vi "Write Evaluations to Limit File.vi"(8 "error in (no error)":errorcluster, 9 "Test Modes":string[](array[string]), 10 "Evaluations In":T1[](array[typedef]) {"Low Limit" format="%#_13g"; "SI Scaling" items=["femto"=-15, "pico"=-12, "nano"=-9, "micro"=-6, "milli"=-3, "percent"=-2, ""=0, "kilo"=3, "mega"=6, "giga"=9, "tera"=12]}, 11 "Limits File Path":path) -> (0 "error out":errorcluster)   [LabVIEW 2018, in "Test Number and Bin Generator.lvlib" / "Test Number and Bin Generator.lvclass"]
uses:
  Test Number and Bin Generator.lvclass
  Plugins/TestStand API Tools (TSAT).lvlibp/Evaluation Actions/Includes/Controls/TSAT Evaluation.ctl
  Plugins/TestStand API Tools (TSAT).lvlibp/Evaluation Actions/Includes/Controls/TSAT Eval SI Unit Scaling.ctl
  Plugins/TestStand API Tools (TSAT).lvlibp/Evaluation Actions/Includes/Controls/TSAT Evaluation Type.ctl
  Plugins/TestStand API Tools (TSAT).lvlibp/Evaluation Actions/TSAT Evaluation Actions.lvlib
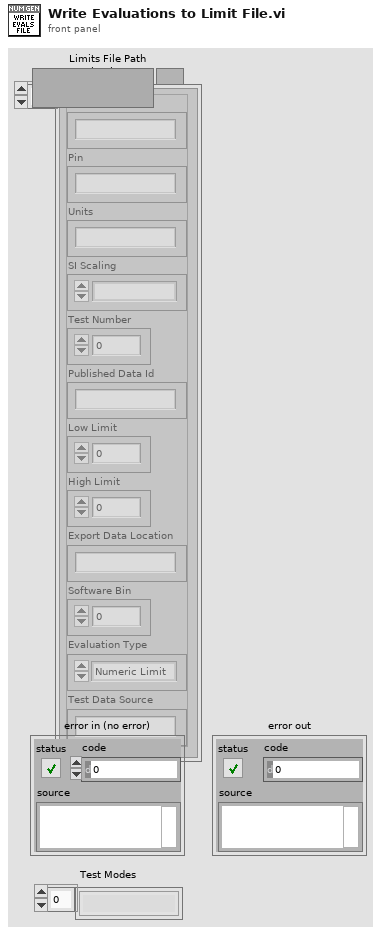
[diagram p1: front panel]
types:
  T1 = typedef "TestStand API Tools (TSAT).lvlibp/TSAT Evaluation Actions.lvlib/TSAT Evaluation.ctl" = cluster{"Test Name":string, "Pin":string, "Units":string, "SI Scaling":T2, "Test Number":i32, "Published Data Id":string, "Low Limit":dbl, "High Limit":dbl, "Export Data Location":string, "Software Bin":i64, "Evaluation Type":T3, "Test Data Source":string}
  T2 = typedef "TestStand API Tools (TSAT).lvlibp/TSAT Evaluation Actions.lvlib/TSAT Eval SI Unit Scaling.ctl" = i16
  T3 = typedef "TestStand API Tools (TSAT).lvlibp/TSAT Evaluation Actions.lvlib/TSAT Evaluation Type.ctl" = enum16{"Numeric Limit", "Pass/Fail", "None"}
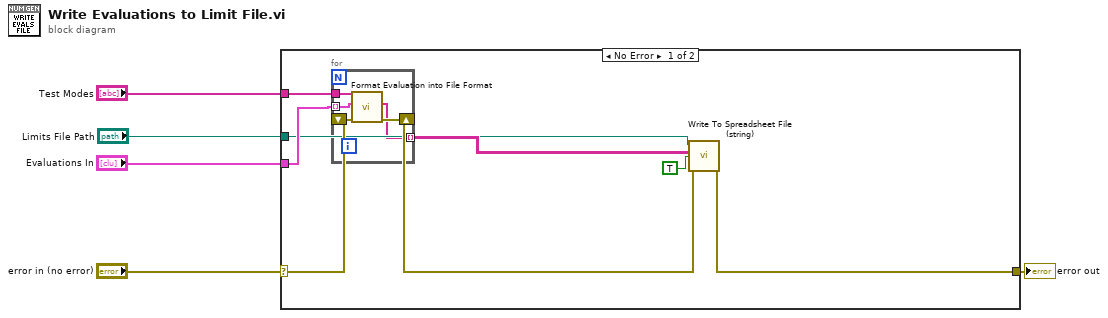
[diagram p0: block diagram]
diagram:
  n1 = case shown="No Error" "error in (no error)" {
    selector: "error in (no error)" -> [w12 w19]
    tunnel: [w13 w19] -> w5
    tunnel: "Evaluations In" -> [w10 _]
    tunnel: "Test Modes" -> [w7 _]
    tunnel: "Limits File Path" -> [w6 _]
    frame No Error {
      n2 = for {
        shift-right: [w17] -> w11
        shift-left: w12 -> [w18]
        tunnel: w10 -> [w16] mode=indexing
        tunnel: [w15] -> w9 mode=indexing
        tunnel: w7 -> [w14]
        n3 = call "Format Evaluation into File Format.vi"("error in (no error)"=w18, "Evaluation"=w16, "Test Modes"=w14) -> ("error out"=w17:errorcluster, "Row Data Out"=w15:string[])  [unwired: 7 in]
      }
      n4 = call "Write To Spreadsheet File (string).vi"("file path (dialog if empty)"=w6, "2D data"=w9, "error in"=w11, "append to file? (new file:F)"=TRUE) -> ("error out"=w13:errorcluster)  [unwired: 5 in, 1 out]
    }
    frame Error {
    }
  }
  "error out" <- w5
